vi "LLB Pre-Build CHM Build.vi"(6 "Top Level/Always Included VIs":path[](array[path]), 7 "Main Destination Path":path, 9 "Target Name":string, 10 "Build Specification Name":string, 11 "Project Path":path) -> (0 "error out":errorcluster)   [LabVIEW 2017]
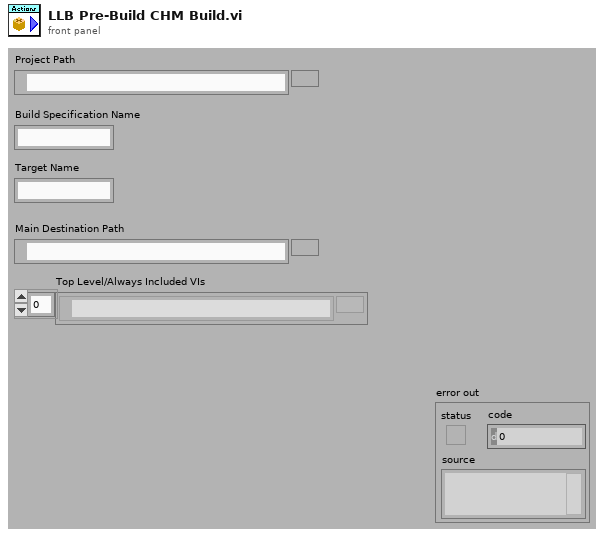
[diagram p1: front panel]
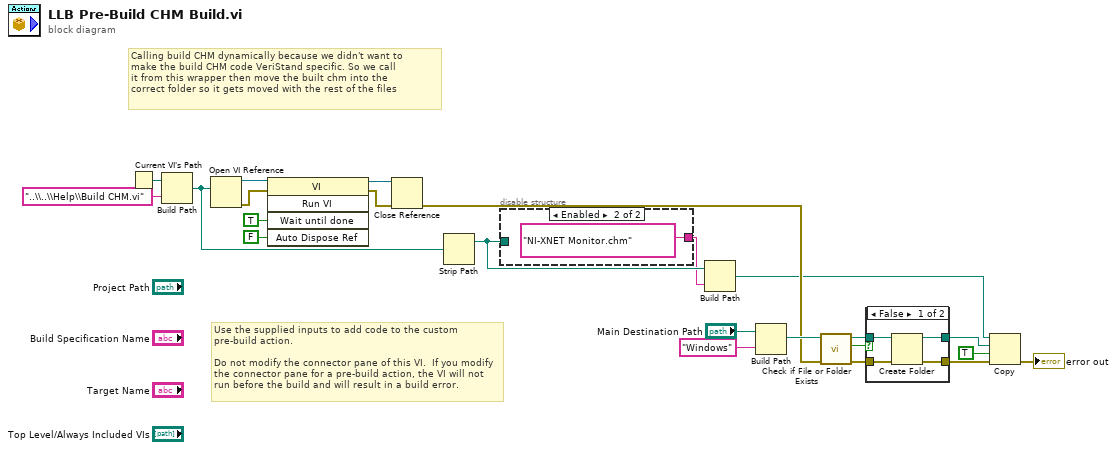
[diagram p0: block diagram]
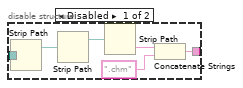
[diagram p2: hidden frame]
diagram:
  # "Calling build CHM dynamically because we didn't want to \nmake the build CHM code VeriStand specific. So we call\nit from this wrapper then move the built chm into the\ncorrect folder so it gets moved with the rest of the files"
  # "Use the supplied inputs to add code to the custom pre-build action.\n\nDo not modify the connector pane of this VI.  If you modify the connector pane for a pre-build action, the VI will not run before the build and will result in a build error."
  n1 = Current VI's Path() -> (path=w23:path)
  n2 = Build Path(base path=w23, name or relative path="..\\..\\Help\\Build CHM.vi") -> (appended path=w15:path)
  n3 = Open VI Reference(vi path=w15) -> (vi reference=w21:refnum<vi>, error out=w20:errorcluster)  [unwired: 5 in]
  n4 = invoke class="VI" method="Run VI"(reference=w21, error in=w20, "Wait until done"=TRUE ("Wait Until Done"), "Auto Dispose Ref"=FALSE ("Auto Dispose Reference")) -> (reference out=w17:refnum<vi>, error out=w16:errorcluster)  [unwired: 1 in, 3 out]
  n5 = Close Reference(reference=w17, error in (no error)=w16) -> (error out=w9:errorcluster)
  n6 = Strip Path(path=w15) -> (stripped path=w14:path)  [unwired: 1 out]
  n7 = disable-structure shown="Enabled" {
    disable-tunnel: w14 -> [w29 _]
    disable-tunnel: [w24 "NI-XNET Monitor.chm"] -> w13
    frame Disabled {
      n8 = Strip Path(path=w29) -> (stripped path=w28:path)  [unwired: 1 out]
      n9 = Strip Path(path=w28) -> (stripped path=w27:path)  [unwired: 1 out]
      n10 = Strip Path(path=w27) -> (name=w26:string)  [unwired: 1 out]
      n11 = Concatenate Strings(w26, ".chm" ("string")) -> (w24:string)
    }
    frame Enabled {
    }
  }
  n12 = Build Path(base path=w14, name or relative path=w13) -> (appended path=w2:path)
  n13 = Build Path(base path="Main Destination Path", name or relative path="Windows") -> (appended path=w10:path)
  n14 = call <vilib>:"Check if File or Folder Exists.vi"("error in (no error)"=w9, "path"=w10) -> ("error out"=w6:errorcluster, "file or folder exists?"=w8:bool, "dup path"=w7:path)  [unwired: 7 in]
  n15 = case shown="False" w8 {
    tunnel: w7 -> [w33 w36]
    tunnel: w6 -> [w34 w35]
    tunnel: [w32 w36] -> w4
    tunnel: [w31 w35] -> w5
    frame False {
      n16 = Create Folder(path (use dialog)=w33, error in=w34) -> (created path=w32:path, error out=w31:errorcluster)  [unwired: 1 in, 1 out]
    }
    frame True {
    }
  }
  n17 = Copy(8:w5, 9:TRUE ("overwrite (F)"), 10:w4, 11:w2) -> (0:→"error out":errorcluster)  [unwired: 1 in, 2 out]
